vi "Update Housekeeping@Write HK Data.vi"(8 "error in (no error)":errorcluster, 10 "HK Data":T1(array[cluster]), 11 "Update Housekeeping MSG in":refnum<class "Update Housekeeping MSG.lvclass">) -> (0 "error out":errorcluster, 3 "Update Housekeeping MSG out":refnum<class "Update Housekeeping MSG.lvclass">)   [LabVIEW 2014, in "eCRDS Library.lvlib" / "Update Housekeeping MSG.lvclass"]
uses:
  Update Housekeeping MSG.lvclass
  Update Housekeeping MSG.lvclass/Update Housekeeping MSG.ctl
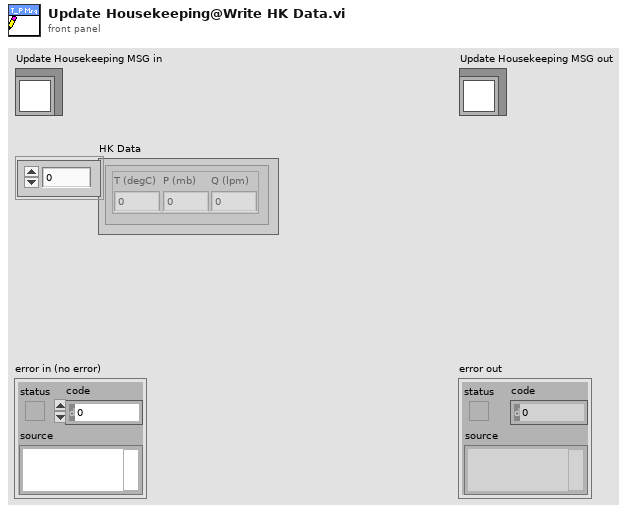
[diagram p1: front panel]
types:
  T1 = cluster{"T (degC)":dbl, "P (mb)":dbl, "Q (lpm)":dbl}[]
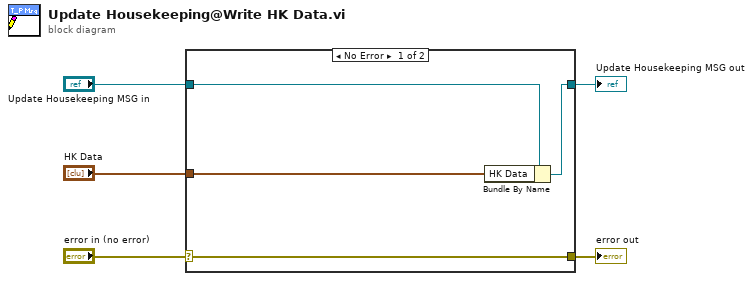
[diagram p0: block diagram]
diagram:
  n1 = case shown="No Error" "error in (no error)" {
    selector: "error in (no error)" -> [w9 w10]
    tunnel: [w9 w10] -> w4
    tunnel: [w7 w11] -> w2
    tunnel: "Update Housekeeping MSG in" -> [w8 w11]
    tunnel: "HK Data" -> [w6 _]
    frame No Error {
      n2 = Bundle By Name(cluster=w8, "HK Data"=w6) -> (w7:refnum<class "Update Housekeeping MSG.lvclass">)
    }
    frame Error {
    }
  }
  "error out" <- w4
  "Update Housekeeping MSG out" <- w2
